vi "LoadImageData.vi"(8 "error in (no error)":errorcluster, 11 "path":path) -> (0 "error out":errorcluster, 3 "image data":T1)   [LabVIEW 2019, in "AnimatorXControl.xctl"]
uses:
  AnimatorXControl.xctl
  <vilib>/picture/picture.llb/imagedata.ctl
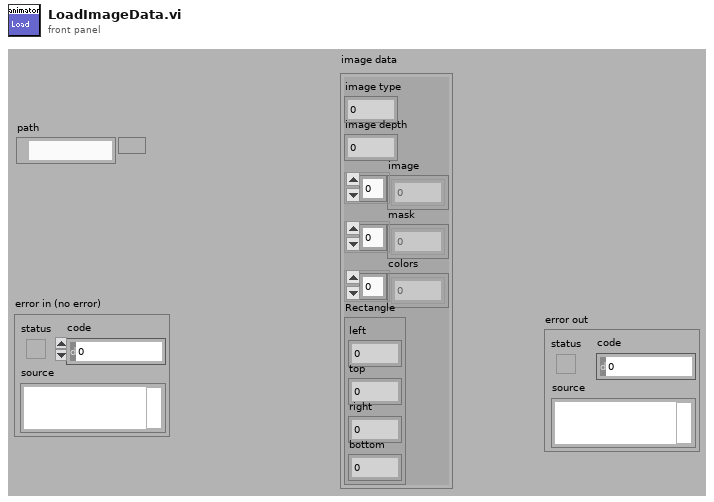
[diagram p1: front panel]
types:
  T1 = typedef "imagedata.ctl" = cluster{"image type":i32, "image depth":i32, "image":u8[], "mask":u8[], "colors":u32[], "Rectangle":cluster{"left":i16, "top":i16, "right":i16, "bottom":i16}}
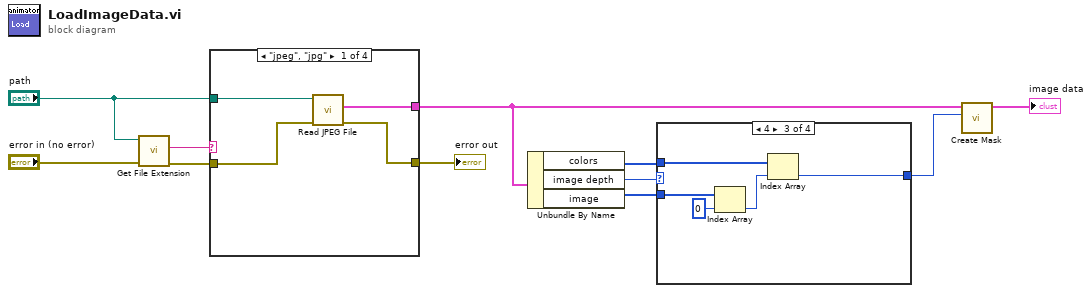
[diagram p0: block diagram]
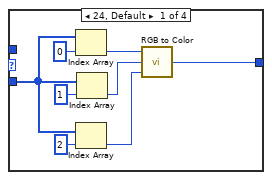
[diagram p2: hidden frame]
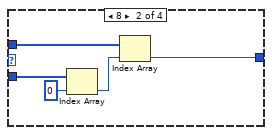
[diagram p3: hidden frame]
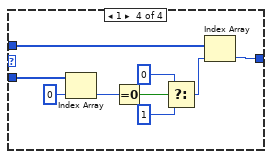
[diagram p4: hidden frame]
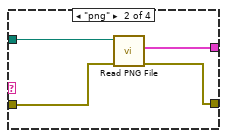
[diagram p5: hidden frame]
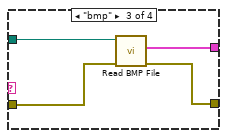
[diagram p6: hidden frame]
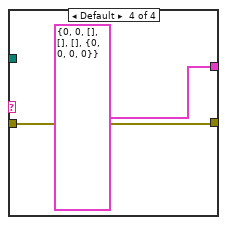
[diagram p7: hidden frame]
diagram:
  n1 = call <vilib>:"Get File Extension.vi"("error in (no error)"="error in (no error)", "file"="path") -> ("error out"=w7:errorcluster, "lowercase file extension"=w9:string)  [unwired: 5 in, 3 out]
  n2 = case shown="\"jpeg\", \"jpg\"" w9 {
    tunnel: w7 -> [w14 w19 w21 w24]
    tunnel: [w13 w18 w23 w24] -> w11
    tunnel: "path" -> [w15 w16 w22 _]
    tunnel: [w12 w17 w20 T1 {"image type"=0, "image depth"=0, "image"=[], "mask"=[], "colors"=[], "Rectangle"={"left"=0, "top"=0, "right"=0, "bottom"=0}} ("image data")] -> w2
    frame "jpeg", "jpg" {
      n3 = call <vilib>:"Read JPEG File.vi"("error in (no error)"=w14, "path to JPEG file"=w15) -> ("error out"=w13:errorcluster, "image data"=w12:T1)  [unwired: 7 in, 1 out]
    }
    frame "png" {
      n4 = call <vilib>:"Read PNG File.vi"("error in (no error)"=w19, "path to PNG file"=w16) -> ("error out"=w18:errorcluster, "image data"=w17:T1)  [unwired: 7 in, 1 out]
    }
    frame "bmp" {
      n5 = call <vilib>:"Read BMP File.vi"("error in (no error)"=w21, "path to BMP file"=w22) -> ("error out"=w23:errorcluster, "image data"=w20:T1)  [unwired: 7 in, 1 out]
    }
    frame Default {
    }
  }
  "error out" <- w11
  n6 = Unbundle By Name(w2) -> ("colors"=w4:u32[], "image depth"=w6:i32, "image"=w5:u8[])
  n7 = case shown="4" w6 {
    tunnel: w5 -> [w29 w38 w43 w52]
    tunnel: w4 -> [_ w36 w41 w48]
    tunnel: [w31 w34 w39 w44] -> w3
    frame 24, Default {
      n8 = Index Array(array=w29, index=0) -> (element=w32:u8)
      n9 = Index Array(array=w29, index=2) -> (element=w26:u8)
      n10 = Index Array(array=w29, index=1) -> (element=w27:u8)
      n11 = call <vilib>:"RGB to Color.vi"("B"=w26, "G"=w27, "R"=w32) -> ("Color"=w31:u32)
    }
    frame 8 {
      n12 = Index Array(array=w38, index=0) -> (element=w35:u8)
      n13 = Index Array(array=w36, index=w35) -> (element=w34:u32)
    }
    frame 4 {
      n14 = Index Array(array=w43, index=0) -> (element=w40:u8)
      n15 = Index Array(array=w41, index=w40) -> (element=w39:u32)
    }
    frame 1 {
      n16 = Index Array(array=w52, index=0) -> (element=w50:u8)
      n17 = Equal To 0?(x=w50) -> (x = 0?=w49:bool)
      n18 = Select(t=u32 0, s=w49, f=u32 1) -> (s? t:f=w45:u32)
      n19 = Index Array(array=w48, index=w45) -> (element=w44:u32)
    }
  }
  n20 = call <vilib>:"Create Mask.vi"("Mask Color (Black)"=w3, "image data"=w2) -> ("image data"=→"image data":T1)  [unwired: 9 in]
